vi "HTTP Get.vi"(3 "Endpoint":string="/Basic/GetStatus", 4 "Port":string="35100", 5 "IP Address":string="10.0.40.83") -> (1 "headers":string, 2 "body":string)   [LabVIEW 2020]
uses:
  <vilib>/httpClient/LabVIEWHTTPClient.lvlib
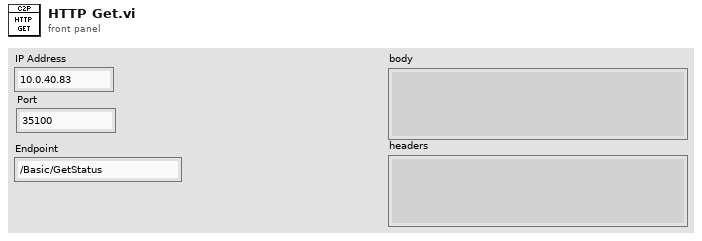
[diagram p1: front panel]
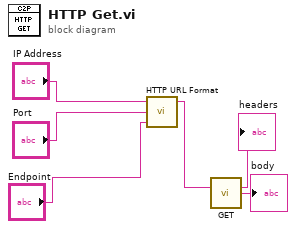
[diagram p0: block diagram]
diagram:
  n1 = call "HTTP URL Format.vi"("Endpoint"="Endpoint", "Port"="Port", "IP Address"="IP Address") -> ("URL"=w1:string)  [unwired: 2 in]
  n2 = call <vilib>:"GET.vi"("url"=w1) -> ("headers"=→"headers":string, "body"=→"body":string)  [unwired: 11 in, 2 out]
